vi "pix.u16.RemapToU32.vi"(5 "ZScale.MarkerValues":cluster{dbl, u32}[](array[cluster]), 8 "img.u16":T1) -> (2 "img.24bit":u32[][](array[numeric]))   [LabVIEW 2020]
uses:
  _controls/img.u16.graph.25pc.axes.ctl
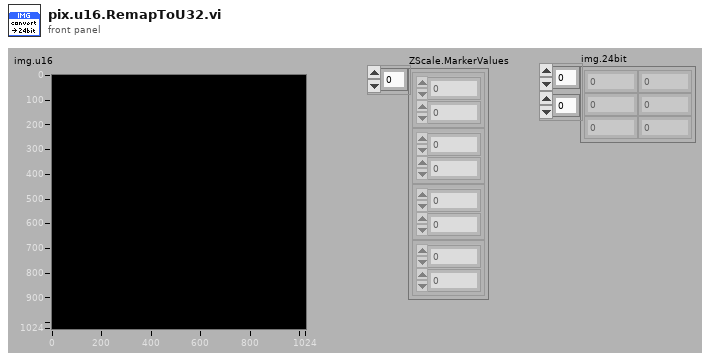
[diagram p1: front panel]
types:
  T1 = typedef "img.u16.graph.25pc.axes.ctl" = u16[][]
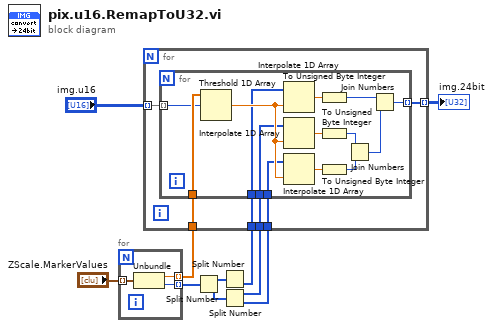
[diagram p0: block diagram]
diagram:
  n1 = for {
    tunnel: "ZScale.MarkerValues" -> [w13] mode=indexing
    tunnel: [w12] -> w2 mode=indexing
    tunnel: [w11] -> w3 mode=indexing
    n2 = Unbundle(w13) -> (w12:dbl, w11:u32)
  }
  n3 = Split Number(x=w3) -> (hi(x)=w5:u16[], lo(x)=w4:u16[])
  n4 = Split Number(x=w5) -> (lo(x)=w6:u8[])  [unwired: 1 out]
  n5 = Split Number(x=w4) -> (hi(x)=w7:u8[], lo(x)=w8:u8[])
  n6 = for {
    tunnel: "img.u16" -> [w19] mode=indexing
    tunnel: [w18] -> w1 mode=indexing
    tunnel: w2 -> [w17]
    tunnel: w8 -> [w16]
    tunnel: w6 -> [w15]
    tunnel: w7 -> [w14]
    n7 = for {
      tunnel: w19 -> [w32] mode=indexing
      tunnel: [w28] -> w18 mode=indexing
      tunnel: w17 -> [w33]
      tunnel: w16 -> [w23]
      tunnel: w15 -> [w25]
      tunnel: w14 -> [w24]
      n8 = Threshold 1D Array(2:w32, 3:w33) -> (0:w31:dbl)  [unwired: 1 out]
      n9 = Interpolate 1D Array(1:w31, 2:w25) -> (0:w26:dbl)
      n10 = Interpolate 1D Array(1:w31, 2:w24) -> (0:w30:dbl)
      n11 = Interpolate 1D Array(1:w31, 2:w23) -> (0:w29:dbl)
      n12 = To Unsigned Byte Integer(number=w26) -> (unsigned 8bit integer=w22:u8)
      n13 = To Unsigned Byte Integer(number=w30) -> (unsigned 8bit integer=w21:u8)
      n14 = To Unsigned Byte Integer(number=w29) -> (unsigned 8bit integer=w20:u8)
      n15 = Join Numbers(hi=w21, lo=w20) -> ((hi.lo)=w27:u16)
      n16 = Join Numbers(hi=w22, lo=w27) -> ((hi.lo)=w28:u32)
    }
  }
  "img.24bit" <- w1
